vi "Configure New Assert Display.vi"(8 "error in (no error)":errorcluster) -> (0 "error out":errorcluster, 2 "Build?":bool, 3 "Assert Display out":refnum<class "Assert Display.lvclass">)   [LabVIEW 2017, in "Assert API Components.lvlib" / "Assert Display.lvlib" / "Assert Display.lvclass"]
doc: "Configures a new assert display."
uses:
  Assert Display.lvclass
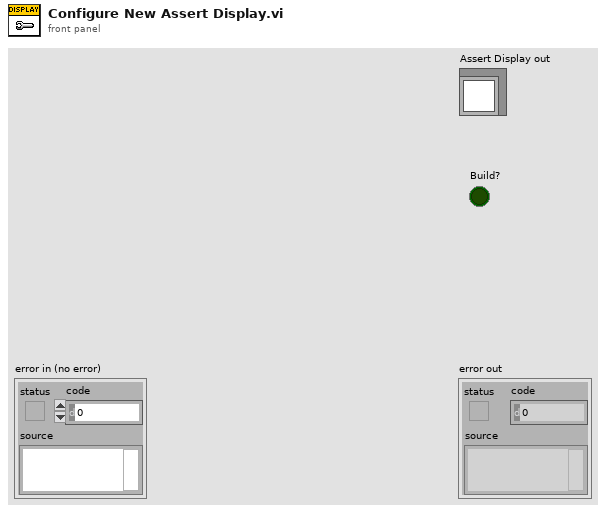
[diagram p1: front panel]
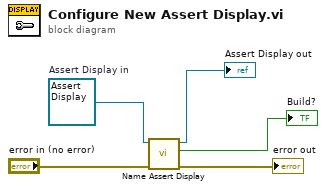
[diagram p0: block diagram]
diagram:
  w3 = refnum<class "Assert Display.lvclass"> refnum  # Assert Display in
  n1 = call "Name Assert Display.vi"("error in (no error)"="error in (no error)", "Assert Display in"=w3) -> ("error out"=→"error out":errorcluster, "Build?"=→"Build?":bool, "Assert Display out"=→"Assert Display out":refnum<class "Assert Display.lvclass">)  [unwired: 7 in]
